vi "2-1 controllo se compreso control.vi"(2 "control":bool, 3 "low limit":dbl(knob) scale=10.0..100.0 scale format="%#_4g", 4 "hight limit":dbl(knob) scale=10.0..100.0 scale format="%#_4g", 5 "data in":dbl format="%.2f") -> (0 "Waveform Chart":dbl(graph), 1 "data out":dbl(knob) scale=0.0..10.0 scale format="%#_4g")   [LabVIEW 2012]
doc: "© Copyright M. Ferrari 1999"
panel:
  # "Se control = ON, bisogna verificare che il valore sia compreso nei limiti\n                     trasferendo il valore di ingresso diviso per il range ( hight limit-low limit)\n                     in uscita; se il valore  \"data in\"  non rientra nei limiti, oppure\nse control = OFF, non viene effettuato nessun controllo e il valore di ingresso passa\n                    direttamente in uscita"
  # "far apparire la scritta ON ,\no la scritta OFF, a seconda\ndei casi, su sfondo bianco"
  # "sostituire con un indicatore \ndi tipo ' meter' con indicatore digitale"
  # "sostituire con due controlli \ndi tipo ' knob' con indicatore digitale"
  # "Eliminare dal pannello tutte le indicazioni in arancio"
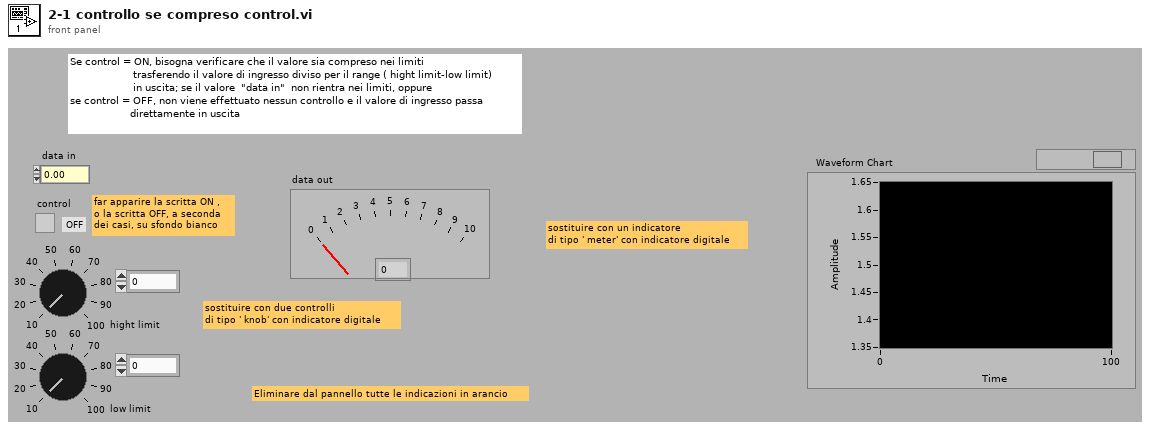
[diagram p1: front panel]
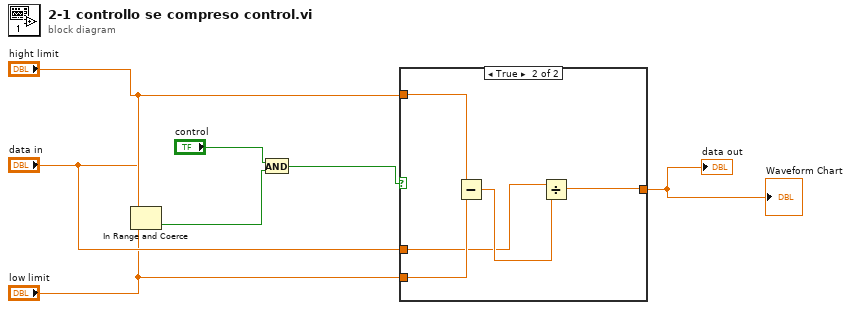
[diagram p0: block diagram]
diagram:
  n1 = In Range and Coerce(upper limit="hight limit", x="data in", lower limit="low limit") -> (In Range?=w6:bool)  [unwired: 1 out]
  n2 = And(x="control", y=w6) -> (x .and. y?=w5:bool)
  n3 = case shown="True" w5 {
    tunnel: "data in" -> [w8 w10]
    tunnel: [w8 w9] -> w4
    tunnel: "hight limit" -> [_ w13]
    tunnel: "low limit" -> [_ w12]
    frame False {
    }
    frame True {
      n4 = Subtract(x=w13, y=w12) -> (x-y=w11:dbl)
      n5 = Divide(x=w10, y=w11) -> (x/y=w9:dbl)
    }
  }
  "data out" <- w4
  "Waveform Chart" <- w4
